vi "Control_verify_voltage.vi"(7 "Timeout (ms)":i32, 8 "에러 입력(에러 없음)":errorcluster, 9 "VTx_Voltage":dbl, 10 "VTxIndex_In":i8, 11 "TCP 네트워크 연결 입력":refnum<k5>) -> (0 "에러 출력":errorcluster, 1 "check_VTx1":dbl, 2 "check_VTx0":dbl, 3 "TCP 네트워크 연결 출력":refnum<k5>, 5 "Verify_voltage":bool)   [LabVIEW 2016]
uses:
  TemperatureMeasure/Thermal_type.vi
panel:
  out "VTx_Selection":dbl
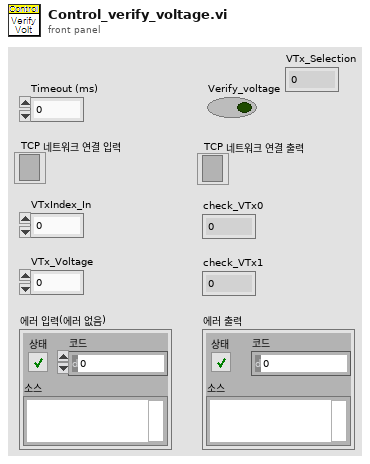
[diagram p1: front panel]
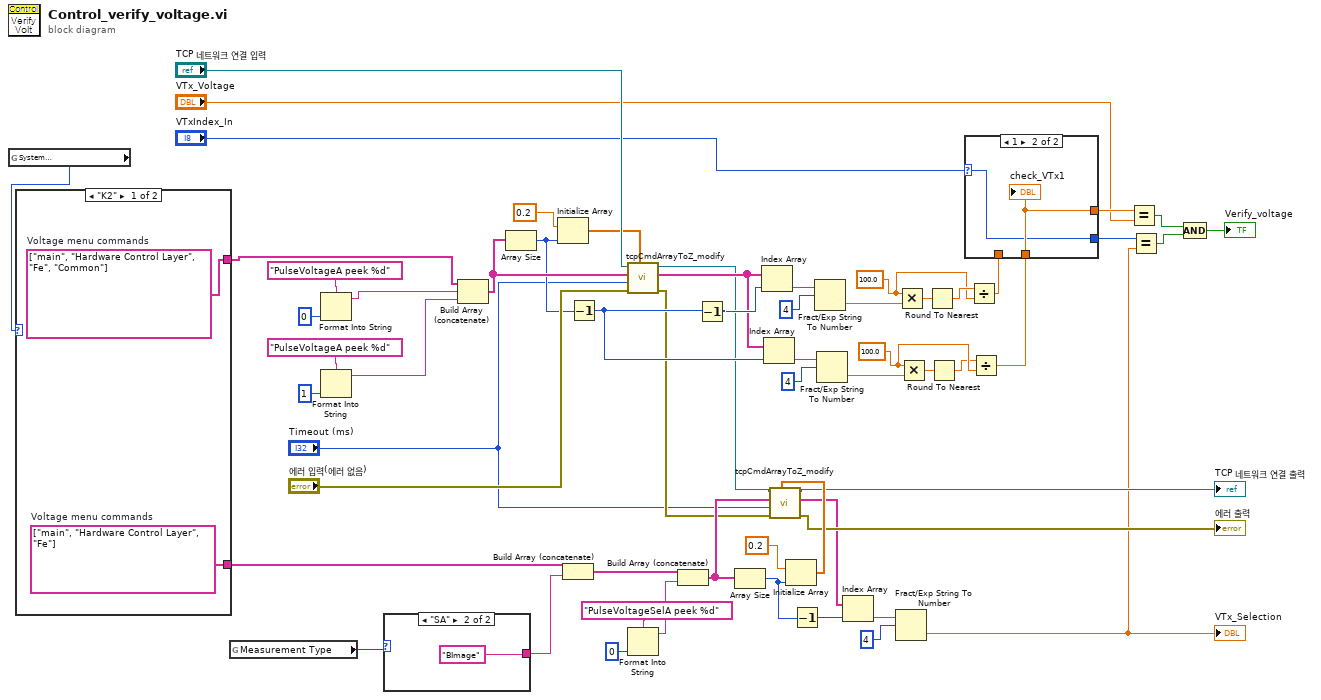
[diagram p0: block diagram]
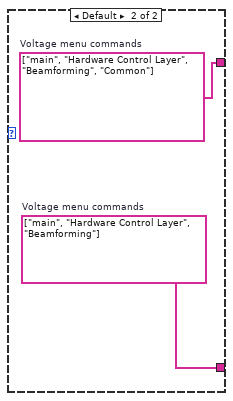
[diagram p2: hidden frame]
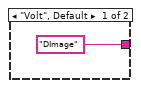
[diagram p3: hidden frame]
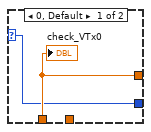
[diagram p4: hidden frame]
diagram:
  w45 = 100.0
  w33 = 100.0
  n1 = global read "Thermal_type.vi" "System \nSelection"() -> (w1:enum32{"Common", "Frosk", "Griffin", "K2"})
  n2 = case shown="\"K2\"" w1 {
    tunnel: [w61 w63] -> w52
    tunnel: [w60 w62] -> w2
    frame "K2" {
      w60 = string[] ["main", "Hardware Control Layer", "Fe"]  # Voltage menu commands
      w61 = string[] ["main", "Hardware Control Layer", "Fe", "Common"]  # Voltage menu commands
    }
    frame Default {
      w62 = string[] ["main", "Hardware Control Layer", "Beamforming"]  # Voltage menu commands
      w63 = string[] ["main", "Hardware Control Layer", "Beamforming", "Common"]  # Voltage menu commands
    }
  }
  n3 = global read "Thermal_type.vi" "Measurement Type"() -> (w26:enum32{"Volt", "SA"})
  n4 = Format Into String(format string="PulseVoltageA peek %d", i8 0 ("입력 1")) -> (resulting string=w39:string)  [unwired: 2 in, 1 out]
  n5 = Format Into String(format string="PulseVoltageA peek %d", i8 1 ("입력 1")) -> (resulting string=w42:string)  [unwired: 2 in, 1 out]
  n6 = case shown="\"SA\"" w26 {
    tunnel: ["DImage" "BImage"] -> w25
    frame "Volt", Default {
    }
    frame "SA" {
    }
  }
  n7 = Build Array (concatenate)(w52, w39, w42) -> (w37:string[])
  n8 = Array Size(array=w37) -> (size(s)=w29:i32)
  n9 = Initialize Array(0.2 ("원소"), w29) -> (w28:dbl[])
  n10 = Build Array (concatenate)(w2, w25) -> (w22:string[])
  n11 = Decrement(x=w29) -> (x-1=w51:i32)
  n12 = call "tcpCmdArrayToZ_modify.vi"("Delay (sec)"=w28, "error in (no error)"="에러 입력(에러 없음)", "Timeout (ms)"="Timeout (ms)", "Command array"=w37, "connection ID in"="TCP 네트워크 연결 입력") -> ("error out"=w16:errorcluster, "Receive array"=w49:string[], "connection ID out"=w17:refnum<k5>)  [unwired: 2 in, 2 out]
  n13 = Format Into String(format string="PulseVoltageSelA peek %d" ("포맷 문자열"), i8 0 ("입력 1")) -> (resulting string=w23:string)  [unwired: 2 in, 1 out]
  n14 = Build Array (concatenate)(w22, w23) -> (w19:string[])
  n15 = Decrement(x=w51) -> (x-1=w50:i32)
  n16 = Array Size(array=w19) -> (size(s)=w13:i32)
  n17 = Index Array(array=w49, index=w50) -> (element=w30:string)
  n18 = Index Array(array=w49, index=w51) -> (element=w48:string)
  n19 = Initialize Array(0.2 ("원소"), w13) -> (w20:dbl[])
  n20 = call "tcpCmdArrayToZ_modify.vi"("Delay (sec)"=w20, "error in (no error)"=w16, "Timeout (ms)"="Timeout (ms)", "Command array"=w19, "connection ID in"=w17) -> ("error out"=→"에러 출력":errorcluster, "Receive array"=w9:string[], "connection ID out"=→"TCP 네트워크 연결 출력":refnum<k5>)  [unwired: 2 in, 2 out]
  n21 = Decrement(x=w13) -> (x-1=w10:i32)
  n22 = Fract/Exp String To Number(string=w30, offset=4 ("오프셋")) -> (number=w35:dbl)  [unwired: 2 in, 1 out]
  n23 = Fract/Exp String To Number(string=w48, offset=4 ("오프셋")) -> (number=w43:dbl)  [unwired: 2 in, 1 out]
  n24 = Index Array(array=w9, index=w10) -> (element=w11:string)
  n25 = Fract/Exp String To Number(string=w11, offset=4 ("오프셋")) -> (number=w7:dbl)  [unwired: 2 in, 1 out]
  "VTx_Selection" <- w7
  n26 = Multiply(x=w33, y=w35) -> (x*y=w32:dbl)
  n27 = Multiply(x=w45, y=w43) -> (x*y=w46:dbl)
  n28 = Round To Nearest(number=w32) -> (nearest integer value=w34:dbl)
  n29 = Round To Nearest(number=w46) -> (nearest integer value=w44:dbl)
  n30 = Divide(x=w34, y=w33) -> (x/y=w54:dbl)
  n31 = Divide(x=w44, y=w45) -> (x/y=w55:dbl)
  n32 = case shown="1" "VTxIndex_In" {
    selector: "VTxIndex_In" -> [w66 w68]
    tunnel: w54 -> [w67 _]
    tunnel: w55 -> [_ w69]
    tunnel: [w67 w69] -> w57
    tunnel: [w66 w68] -> w8
    frame 0, Default {
      "check_VTx0" <- w67
    }
    frame 1 {
      "check_VTx1" <- w69
    }
  }
  n33 = Equal?(x=w57, y="VTx_Voltage") -> (x = y?=w6:bool)
  n34 = Equal?(x=w8, y=w7) -> (x = y?=w5:bool)
  n35 = Compound Arithmetic op=AND(w6, w5) -> (→"Verify_voltage":bool)
